vi "MAG OFF.vi"(0 "VISA Resource Name Out":refnum<visa-resource-name>, 5 "MagQ":refnum<queue>, 7 "Boolean":bool, 9 "PSU Status Out":T1 {"Trip Current" format="%.3f"; "Trip Field" format="%.4f"; "Voltage" format="%.2f"; "Field Constant" format="%.6f"; "MID Setpoint (T)" format="%.4f"; "MID Setpoint (A)" format="%.3f"; "MAX Setpoint (T)" format="%.4f"; "MAX Setpoint (A)" format="%.3f"; "Heater Voltage" format="%.2f"; "V Limit (V)" format="%.2f"; "Ramp Rate (A/s)" format="%.3f"; "Output (A)" format="%.3f"; "Output (T)" format="%.4f"; "Persistent Current" format="%.3f"; "Persistent Field" format="%.4f"}, 11 "Error out":errorcluster) -> (4 "VISA Resource Name Out 2":refnum<visa-resource-name>, 6 "MagQ 2":refnum<queue>, 8 "Boolean 2":bool, 10 "PSU Status Out 2":T1 {"Trip Current" format="%.3f"; "Trip Field" format="%.4f"; "Voltage" format="%.2f"; "Field Constant" format="%.6f"; "MID Setpoint (T)" format="%.4f"; "MID Setpoint (A)" format="%.3f"; "MAX Setpoint (T)" format="%.4f"; "MAX Setpoint (A)" format="%.3f"; "Heater Voltage" format="%.2f"; "V Limit (V)" format="%.2f"; "Ramp Rate (A/s)" format="%.3f"; "Output (A)" format="%.3f"; "Output (T)" format="%.4f"; "Persistent Current" format="%.3f"; "Persistent Field" format="%.4f"}, 15 "error out":errorcluster)   [LabVIEW 2025]
uses:
  <instrlib>/SMS LabVIEW Drivers/Source Code/Cryogenic Ltd SMSXXX.lvlib
  <instrlib>/SMS LabVIEW Drivers/Source Code/Public/PSU Status.ctl
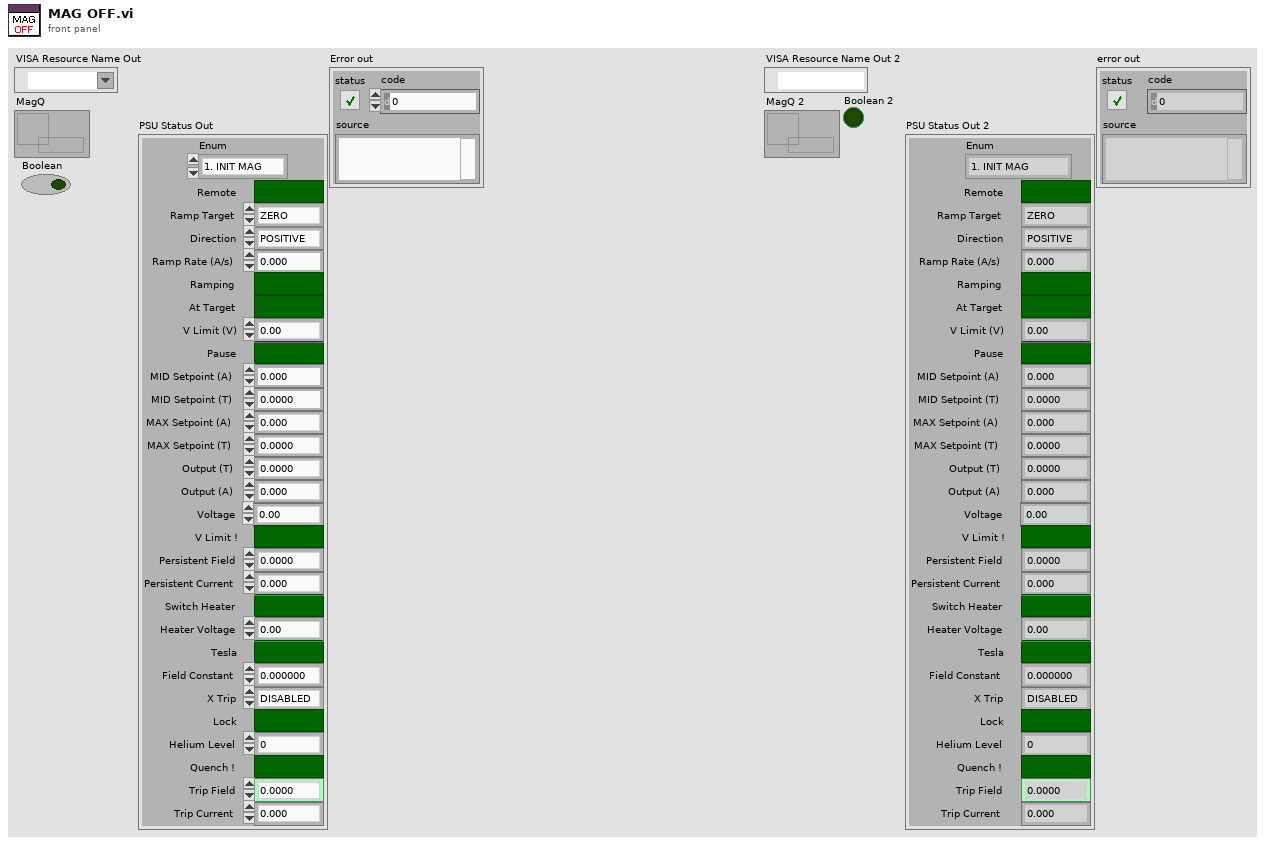
[diagram p1: front panel]
types:
  T1 = typedef "Cryogenic Ltd SMSXXX.lvlib/PSU Status.ctl" = cluster{"Ramp Target":enum16{"ZERO", "MID", "MAX"}, "Pause":bool, "Switch Heater":bool, "Persistent Field":dbl, "Persistent Current":dbl, "Tesla":bool, "Output (T)":dbl, "Output (A)":dbl, "X Trip":enum16{"DISABLED", "ENABLED", "ACTIVE"}, "Ramp Rate (A/s)":dbl, "V Limit (V)":dbl, "Heater Voltage":dbl, "MAX Setpoint (A)":dbl, "MAX Setpoint (T)":dbl, "MID Setpoint (A)":dbl, "MID Setpoint (T)":dbl, "Lock":bool, "Field Constant":dbl, "Remote":bool, "Direction":enum16{"POSITIVE", "NEGATIVE", "OPEN", "UNIPOLAR"}, "Helium Level":u16, "Quench !":bool, "Voltage":dbl, "V Limit !":bool, "Ramping":bool, "At Target":bool, "Trip Field":dbl, "Trip Current":dbl, "Enum":enum16{"1. INIT MAG", "2. MAG ON ", "3. MAG_STAB", "4. MAG IDLE", "5. NEXT FIELD", "6. MAG OFF (Reset)"}}
  T2 = enum16{"1. INIT MAG", "2. MAG ON", "3. MAG_STAB", "4. MAG IDLE", "5. PREP NEXT FIELD", "6. APPLY NEXT FIELD", "7. PREP OFF", "8. MAG OFF (Reset)"}
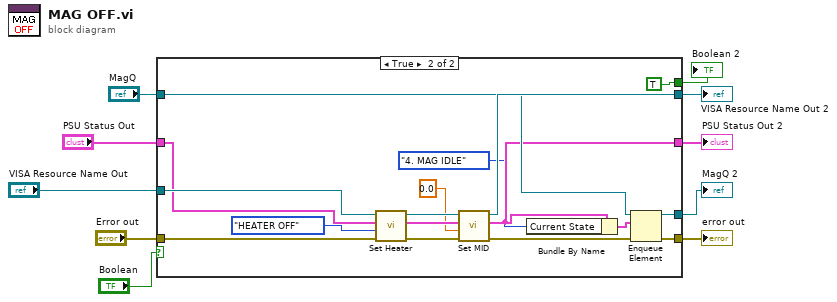
[diagram p0: block diagram]
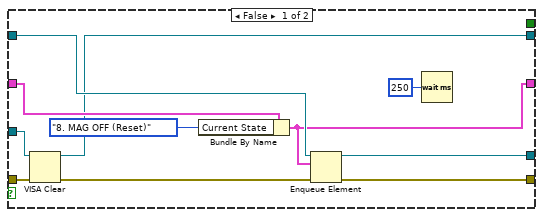
[diagram p2: hidden frame]
diagram:
  n1 = case shown="True" "Boolean" {
    tunnel: "VISA Resource Name Out" -> [w16 w37]
    tunnel: "PSU Status Out" -> [w20 w36]
    tunnel: "Error out" -> [w15 w35]
    tunnel: [_ TRUE] -> w1
    tunnel: [w12 w26] -> w5
    tunnel: [w14 w29] -> w6
    tunnel: [w17 w22] -> w3
    tunnel: "MagQ" -> [w21 w28]
    tunnel: [w18 w24] -> w4
    frame False {
      n2 = VISA Clear(VISA resource name=w16, error in (no error)=w15) -> (VISA resource name out=w14:refnum<visa-resource-name>, error out=w13:errorcluster)
      n3 = Bundle By Name(cluster=w20, "Current State"=T2."8. MAG OFF (Reset)") -> (w12:T1)
      n4 = Enqueue Element(queue=w21, element=w12, error in (no error)=w13) -> (queue out=w18:refnum<queue>, error out=w17:errorcluster)  [unwired: 1 in, 1 out]
      n5 = Wait (ms)(milliseconds to wait=u32 250) -> ()  [unwired: 1 out]
    }
    frame True {
      n6 = call <instrlib>:"Set Heater.vi"("Error in (no error)"=w35, "Heater (On/Off)"=enum16{"HEATER OFF", "HEATER ON"}."HEATER OFF", "PSU Status In"=w36, "VISA Resource Name In"=w37) -> ("Error out"=w32:errorcluster, "PSU Status Out"=w31:T1, "VISA Resource Name Out"=w33:refnum<visa-resource-name>)  [unwired: 4 in, 1 out]
      n7 = call <instrlib>:"Set MID.vi"("Error in (no error)"=w32, "MID (T or A)"=0.0, "PSU Status In"=w31, "VISA Resource Name In"=w33) -> ("Error out"=w23:errorcluster, "PSU Status Out"=w26:T1, "VISA Resource Name Out"=w29:refnum<visa-resource-name>)  [unwired: 4 in, 1 out]
      n8 = Bundle By Name(cluster=w26, "Current State"=T2."4. MAG IDLE") -> (w27:T1)
      n9 = Enqueue Element(queue=w28, element=w27, error in (no error)=w23) -> (queue out=w24:refnum<queue>, error out=w22:errorcluster)  [unwired: 1 in, 1 out]
    }
  }
  "VISA Resource Name Out 2" <- w6
  "PSU Status Out 2" <- w5
  "MagQ 2" <- w4
  "error out" <- w3
  "Boolean 2" <- w1
